vi "FTW-Actor-Destroy.vi"(0 "FTW Actor Instance":refnum<class "FTW-ActorInstance.lvclass">, 5 "Force Destroy?":bool=TRUE, 11 "error in":errorcluster) -> (15 "error out":errorcluster)   [LabVIEW 2013, in "FTW-ActorInstance.lvclass"]
uses:
  FTW-ActorInstance.lvclass
  FTW-Actor-FrameworkEvent.ctl
  FTW-ActorInstance.lvclass/FTW-ActorInstance.ctl
  EventLogger/FTW-Logger.lvclass
  Core/src/Error/FTW-ERR-Clear.vi
  JobSequencer/FTW-JobSequencer.lvclass
  Router/FTW-Router.lvclass
  Publisher/FTW-Publisher.lvclass
panel:
  # "Inputs"
  # "Outputs"
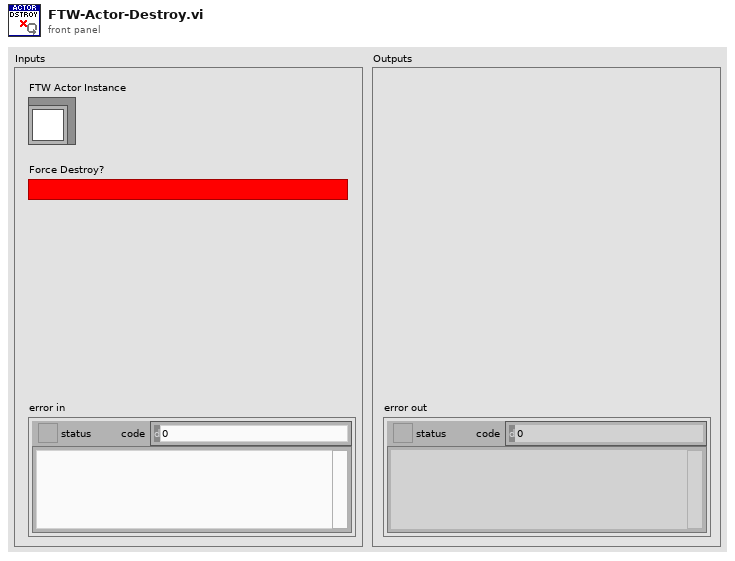
[diagram p1: front panel]
types:
  T1 = typedef "FTW-ActorInstance.lvclass/FTW-Actor-FrameworkEvent.ctl" = enum16{"Instance Initializing", "Instance Initialized", "Instance Job", "Instance Handle Request", "Instance Shutting Down", "Instance Destroyed"}
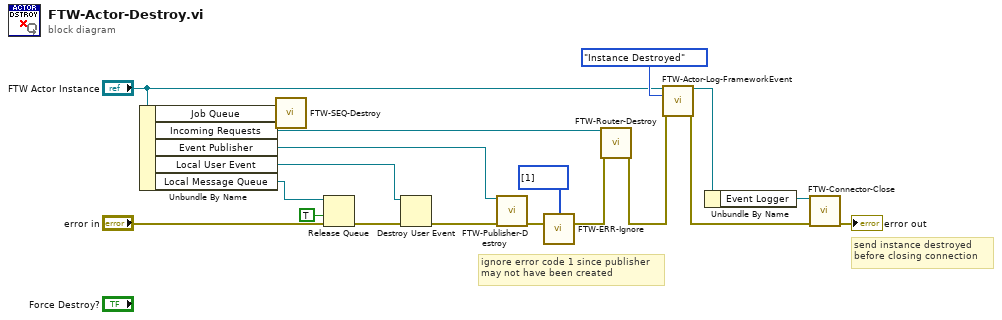
[diagram p0: block diagram]
diagram:
  # "ignore error code 1 since publisher\nmay not have been created"
  # "send instance destroyed\nbefore closing connection"
  n1 = Unbundle By Name("FTW Actor Instance") -> ("Job Queue"=w19:refnum<class "FTW-JobSequencer.lvclass">, "Incoming Requests"=w18:refnum<class "FTW-Router.lvclass">, "Event Publisher"=w17:refnum<class "FTW-Publisher.lvclass">, "Local User Event"=w4:refnum<user-event>, "Local Message Queue"=w1:refnum<queue>)
  n2 = call "FTW-SEQ-Destroy.vi"("FTW Job Sequencer"=w19) -> ()  [unwired: 1 in]
  n3 = Release Queue(queue=w1, force destroy? (F)=TRUE, error in (no error)="error in") -> (error out=w3:errorcluster)  [unwired: 2 out]
  n4 = Destroy User Event(user event=w4, error in=w3) -> (error out=w5:errorcluster)
  n5 = call "FTW-Publisher-Destroy.vi"("FTW-Publisher In"=w17, "error in"=w5) -> ("error out"=w16:errorcluster)  [unwired: 13 in]
  n6 = call "FTW-ERR-Ignore.vi"("Codes to filter"=i32[] [1], "error to filter"=w16) -> ("filtered error"=w8:errorcluster)  [unwired: 13 in]
  n7 = call "FTW-Router-Destroy.vi"("FTW-Router In"=w18, "error in"=w8) -> ("error out"=w7:errorcluster)  [unwired: 13 in]
  n8 = call "FTW-Actor-Log-FrameworkEvent.vi"("FTW Actor Instance"="FTW Actor Instance", "Framework Event"=FTW-Actor-FrameworkEvent."Instance Destroyed", "error in"=w7) -> ("FTW Actor Instance out"=w10:refnum<class "FTW-ActorInstance.lvclass">, "error out"=w12:errorcluster)  [unwired: 11 in]
  n9 = Unbundle By Name(w10) -> ("Event Logger"=w9:refnum<class "FTW-Logger.lvclass">)
  n10 = call-dynamic "FTW-Connector-Close.vi"("FTW Actor Connector"=w9, "error in"=w12) -> ("error out"=→"error out":errorcluster)  [unwired: 13 in]
